vi "FlatToRichni_measurementlink_measurement_v2_MeasureRequest.vi"(5 "OutputClusterType":T1, 11 "InputCluster":T4) -> (3 "OutputCluster":T1)   [LabVIEW 2020, in "Measurement Service Client V2.lvlib"]
uses:
  Measurement Service Client V2.lvlib
  ni_measurementlink_measurement_v2_MeasureRequest_Flat.ctl
  google_protobuf_Any_Flat.ctl
  ni_measurementlink_PinMapContext_Flat.ctl
  ni_measurementlink_measurement_v2_MeasureRequest.ctl
  google_protobuf_Any.ctl
  ni_measurementlink_PinMapContext.ctl
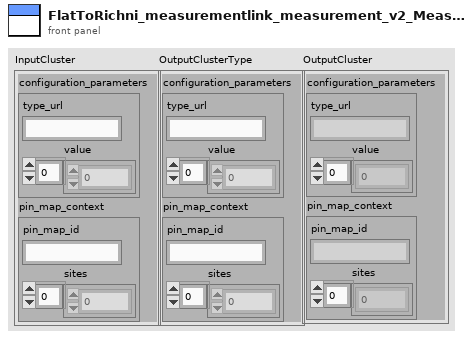
[diagram p1: front panel]
types:
  T1 = typedef "Measurement Service Client V2.lvlib/ni_measurementlink_measurement_v2_MeasureRequest.ctl" = cluster{"configuration_parameters":T2, "pin_map_context":T3}
  T2 = typedef "Measurement Service Client V2.lvlib/google_protobuf_Any.ctl" = cluster{"type_url":string, "value":u8[]}
  T3 = typedef "Measurement Service Client V2.lvlib/ni_measurementlink_PinMapContext.ctl" = cluster{"pin_map_id":string, "sites":i32[]}
  T4 = typedef "Measurement Service Client V2.lvlib/ni_measurementlink_measurement_v2_MeasureRequest_Flat.ctl" = cluster{"configuration_parameters":T5, "pin_map_context":T6}
  T5 = typedef "Measurement Service Client V2.lvlib/google_protobuf_Any_Flat.ctl" = cluster{"type_url":string, "value":u8[]}
  T6 = typedef "Measurement Service Client V2.lvlib/ni_measurementlink_PinMapContext_Flat.ctl" = cluster{"pin_map_id":string, "sites":i32[]}
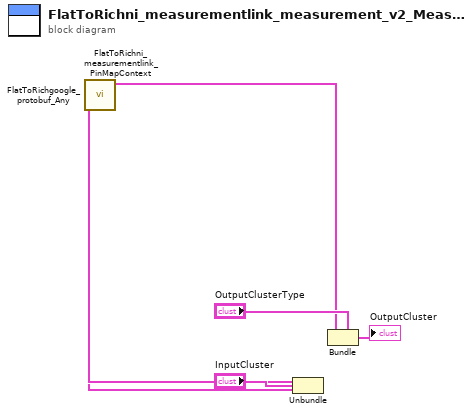
[diagram p0: block diagram]
diagram:
  n1 = Unbundle "Unbundle"("InputCluster") -> ("configuration_parameters"=w4:T5, "pin_map_context"=w2:T6)
  n2 = call "FlatToRichni_measurementlink_PinMapContext.vi"("InputCluster"=w2) -> ("OutputCluster"=w1:T3)  [unwired: 10 in]
  n3 = call "FlatToRichgoogle_protobuf_Any.vi"("InputCluster"=w4) -> ("OutputCluster"=w3:T2)  [unwired: 10 in]
  n4 = Bundle "Bundle"(cluster="OutputClusterType", "configuration_parameters"=w3, "pin_map_context"=w1) -> (→"OutputCluster":T1)
